vi "Write PARmodified.vi"(8 "error in (no error)":errorcluster, 10 "modified (0)":u8, 11 "PAR in":T1) -> (0 "error out":errorcluster, 3 "PAR out":T1)   [LabVIEW 2019, in "Inputs.lvlib"]
uses:
  Inputs.lvlib
  Ctl/Param.ctl
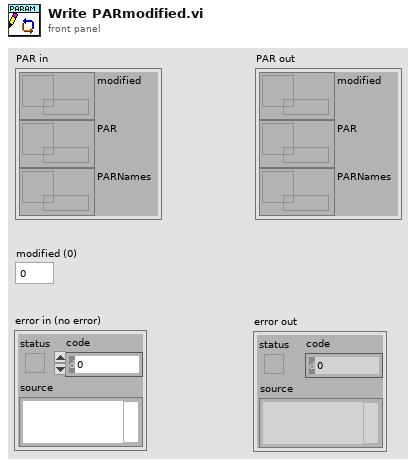
[diagram p1: front panel]
types:
  T1 = typedef "Inputs.lvlib/Param.ctl" = cluster{"modified":refnum<data-value>, "PAR":refnum<data-value>, "PARNames":refnum<data-value>}
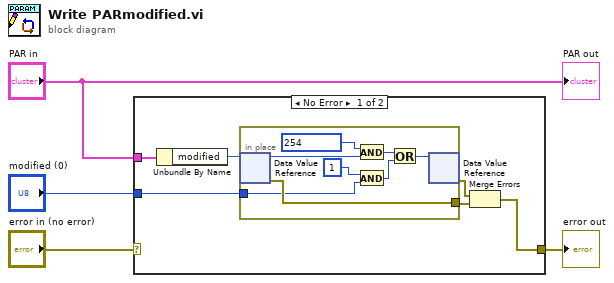
[diagram p0: block diagram]
diagram:
  n1 = case shown="No Error" "error in (no error)" {
    selector: "error in (no error)" -> [_ w19]
    tunnel: [w10 w19] -> w3
    tunnel: "PAR in" -> [w9 _]
    tunnel: "modified (0)" -> [w5 _]
    frame No Error {
      n2 = Unbundle By Name(w9) -> ("modified"=w8:refnum<data-value>)
      n3 = in-place {
        in-place-border: w5 -> [w13]
        in-place-border: [w18] -> w7
        n4 = in-place-dvr #1(w8) -> (w15:u8, w18:errorcluster)
        n5 = And(x=u8 254, y=w15) -> (x .and. y?=w17:u8)
        n6 = And(x=u8 1, y=w13) -> (x .and. y?=w12:u8)
        n7 = Or(x=w17, y=w12) -> (x .or. y?=w11:u8)
        n8 = in-place-dvr #1(w11) -> (w6:errorcluster)  [unwired: 1 out]
      }
      n9 = Merge Errors(w6, w7) -> (w10:errorcluster)
    }
    frame Error {
    }
  }
  "error out" <- w3
  "PAR out" <- "PAR in"
